vi "NetComm_getMatchTime.vi"(8 "error in (no error)":errorcluster) -> (0 "error out":errorcluster, 2 "Match Time":sgl)   [LabVIEW 2017]
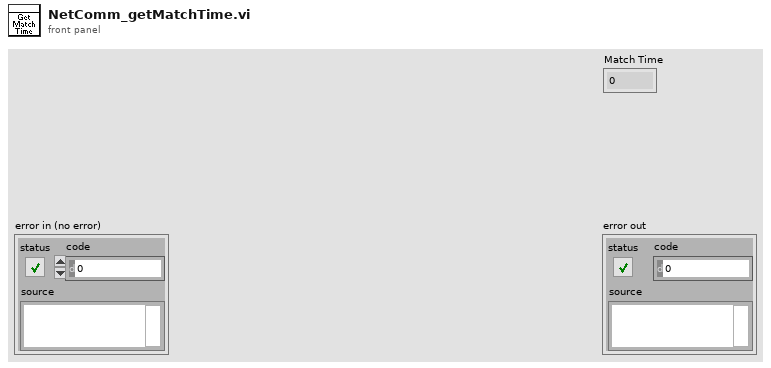
[diagram p1: front panel]
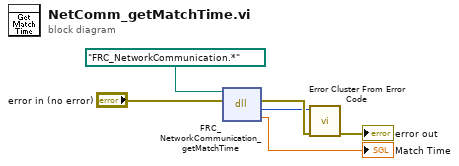
[diagram p0: block diagram]
diagram:
  n1 = dll-call lib="?" fn="FRC_NetworkCommunication_getMatchTime"(path in=path "FRC_NetworkCommunication.*", error in="error in (no error)") -> (error out=w4:errorcluster, "return type"=w3:i32, "matchTime"=→"Match Time":sgl)  [unwired: 2 in, 1 out]
  n2 = call <vilib>:"Error Cluster From Error Code.vi"("error in (no error)"=w4, "error code (0)"=w3) -> ("error out"=→"error out":errorcluster)  [unwired: 7 in]
